vi "Zaber move 1 step.vi"(5 "Maximum":i32, 6 "Direction":enum16{"Forward", "Backward"}(ring), 7 "Device Number":u8, 8 "error in (no error)":errorcluster, 9 "Current position in":i64, 10 "Step Size":i32, 11 "VISA Refnum in":refnum<visa-resource-name>) -> (0 "error out":errorcluster, 2 "Current position out":i64, 3 "VISA Refnum out":refnum<visa-resource-name>)   [LabVIEW 2013]
uses:
  <instrlib>/ZaberTSeries/ZaberTSeries.lvlib
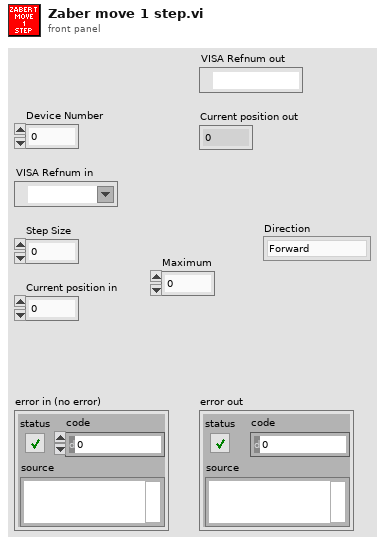
[diagram p1: front panel]
types:
  T1 = cluster{"Device Number":u8, "Command":u8, "Step Size":i32, "Response Count":i32}
  T2 = typedef "ZaberTSeries.lvlib/Response.ctl" = cluster{"Device Number":u8, "Command":u8, "Data":i32}
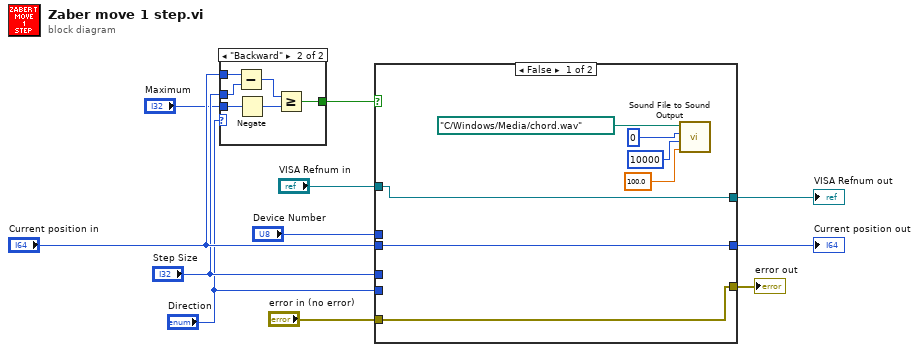
[diagram p0: block diagram]
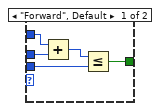
[diagram p2: hidden frame]
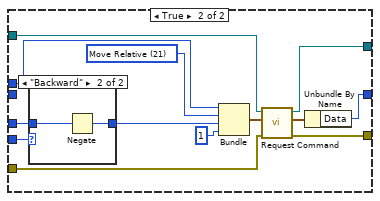
[diagram p3: hidden frame]
diagram:
  n1 = case shown="\"Backward\"" "Direction" {
    tunnel: "Current position in" -> [w13 w22]
    tunnel: [w14 w21] -> w8
    tunnel: "Step Size" -> [w15 w18]
    tunnel: "Maximum" -> [w12 w17]
    frame "Forward", Default {
      n2 = Add(x=w13, y=w15) -> (x+y=w16:i64)
      n3 = Less Or Equal?(x=w16, y=w12) -> (x <= y?=w14:bool)
    }
    frame "Backward" {
      n4 = Subtract(x=w22, y=w18) -> (x-y=w19:i64)
      n5 = Negate(x=w17) -> (-x=w20:i32)
      n6 = Greater Or Equal?(x=w19, y=w20) -> (x >= y?=w21:bool)
    }
  }
  n7 = case shown="False" w8 {
    tunnel: "Step Size" -> [_ w38]
    tunnel: "VISA Refnum in" -> [w24 w37]
    tunnel: [w29 w36] -> w3
    tunnel: [w24 w35] -> w5
    tunnel: "error in (no error)" -> [w29 w33]
    tunnel: [w23 w32] -> w9
    tunnel: "Device Number" -> [_ w31]
    tunnel: "Current position in" -> [w23 _]
    tunnel: "Direction" -> [_ w30]
    frame False {
      n8 = call "Sound File to Sound Output.vi"("Volume"=100.0, "Number of Samples/Iteration"=10000, "Device ID"=u32 0, "File Path"=path "C:/Windows/Media/chord.wav") -> ()
    }
    frame True {
      w39 = u8 21 items=["Echo"=55, "Home"=1, "Move Absolute"=20, "Move Relative"=21, "Move at Constant Speed"=22, "Renumber"=2, "Restore Settings"=36, "Stop"=23] ("Command")
      n9 = case shown="\"Backward\"" w30 {
        tunnel: [w43 w45] -> w42
        tunnel: w38 -> [w43 w44]
        frame "Forward", Default {
        }
        frame "Backward" {
          n10 = Negate(x=w44) -> (-x=w45:i32)
        }
      }
      n11 = Bundle("Device Number"=w31, "Command"=w39, "Step Size"=w42, "Response Count"=1) -> (w41:T1)  [unwired: 1 in]
      n12 = call <instrlib>:"Request Command.vi"("error in (no error)"=w33, "Request"=w41, "VISA resource name"=w37) -> ("error out"=w36:errorcluster, "First Response"=w34:T2, "VISA resource name out"=w35:refnum<visa-resource-name>)  [unwired: 5 in, 1 out]
      n13 = Unbundle By Name(w34) -> ("Data"=w32:i32)
    }
  }
  "Current position out" <- w9
  "VISA Refnum out" <- w5
  "error out" <- w3
